vi "receiver.vi"() -> ()   [LabVIEW 2018]
panel:
  in  "stop":bool
  out "Waveform Graph":waveform(dbl)[](graph)
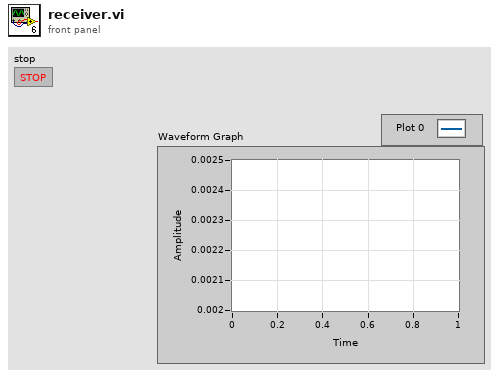
[diagram p1: front panel]
types:
  T1 = enum16{"Read", "Write", "ReadWrite", "BufferedRead", "BufferedReadWrite"}
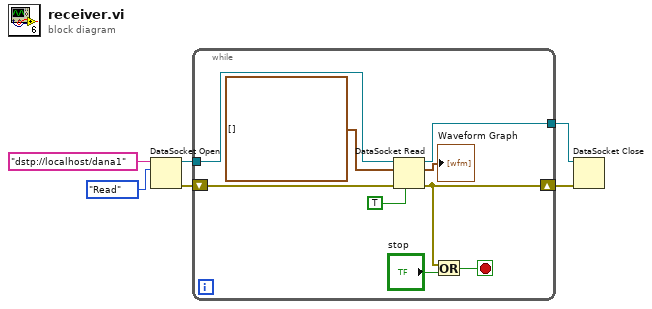
[diagram p0: block diagram]
diagram:
  n1 = DataSocket Open(10:T1."Read" ("mode"), 11:"dstp://localhost/dana1" ("URL")) -> (0:w2:errorcluster, 3:w4:refnum<k13>)  [unwired: 2 in]
  n2 = while {
    tunnel: w4 -> [w12]
    tunnel: [w14] -> w1
    shift-right: [w7] -> w3
    shift-left: w2 -> [w15]
    stop <- w13 stop-if-true
    n3 = DataSocket Read(6:TRUE ("wait for updated value (T)"), 8:w15, 10:waveform(dbl)[] [] ("data"), 11:w12) -> (0:w7:errorcluster, 2:→"Waveform Graph":waveform(dbl)[], 3:w14:refnum<k13>)  [unwired: 1 in, 4 out]
    n4 = Or(x=w7, y="stop") -> (x .or. y?=w13:bool)
  }
  n5 = DataSocket Close(8:w3, 11:w1) -> ()  [unwired: 1 in, 2 out]
